vi "transmit_receive.vi"(4 "samples per readout":i32=5000, 5 "rotary queue":refnum<queue>, 6 "Continious mode":bool, 7 "Enable rotary encoder":bool, 8 "Waveform shift":waveform(dbl), 9 "Waveform drive":waveform(dbl), 10 "channel input for max readouts":T1, 11 "measurement queue":refnum<queue>) -> ()   [LabVIEW 2019]
doc: "This VI is responsible for collecting the data of the MPI experiment from the DAQ and it writes the data of the output waveforms to the DAQ. Generally, this VI can be operated in two modes: Continuous or non-continuous mode. In non-continuous mode, a finite number of samples is read from the ADC and a finite number of samples is written to the DAC. After playing these waveforms and acquiring the samples, the VI stops. The number of samples is determined by the product of \"samples per readout\" and the \"max readouts\" number passed to the VI via a channel structure. The latter allows to update the stopping condition while the acquisition is already running. Acquired data is written to a queue (has to be provided as an input) from which the main VI can then dequeue the readout buckets. Therefore, the sub-VI can be seen as the producer loop while the consumer loop is located in the main VI.\nIn continuous mode, a finite waveform sample is repeated over and over until the data acquisition reaches the set limit or it is stopped. \nInternally, the VI has three different DAQ tasks: Analog input acquisition, analog output generation and digital input acquisition. The analog input acquisition task is the \"master task\" and all other tasks are triggered when the analog data acquisition starts. \nMost of the DAQ settings are read from the global variables (including channel, channel type and sampling rate).\nThe rotary position is taken in the middle of the readout bucket. \nFor safety reasons, the VI ensures that zeros are written to the DAQ when stopping the VI properly."
uses:
  <extravilib>/ChannelInstances/Tag-dbl/))Channel.ctl
  <vilib>/DAQmx/write.llb/DAQmx Write (Analog 1D Wfm NChan NSamp).vi
  <vilib>/DAQmx/read.llb/DAQmx Read (Digital 1D U32 NChan 1Samp).vi
  <vilib>/DAQmx/read.llb/DAQmx Read (Analog 1D Wfm NChan NSamp).vi
  <vilib>/DAQmx/write.llb/DAQmx Write (Analog 2D DBL NChan NSamp).vi
  <vilib>/Waveform/WDTOps.llb/WDT Number of Waveform Samples DBL.vi
  global_variables.vi
  <vilib>/DAQmx/create/channels.llb/DAQmx Create Channel (AO-Voltage-Basic).vi
  <extravilib>/ChannelInstances/Tag-dbl/EndpointRead.vi
  <vilib>/DAQmx/configure/timing.llb/DAQmx Timing (Sample Clock).vi
  <vilib>/DAQmx/create/channels.llb/DAQmx Create Channel (AI-Voltage-Basic).vi
  <vilib>/DAQmx/configure/trigger.llb/DAQmx Start Trigger (None).vi
  <vilib>/DAQmx/configure/trigger.llb/DAQmx Start Trigger (Digital Edge).vi
  <vilib>/DAQmx/miscellaneous.llb/DAQmx Fill In Error Info.vi
  <vilib>/DAQmx/create/channels.llb/DAQmx Create Channel (DI-Digital Input).vi
  <extravilib>/ChannelInstances/Tag-dbl.lvlib
  <resource>/objmgr/daqmx.rc
panel:
  out "Homing & trigger readout":bool[](array[boolean])
  out "sample rate rotary encoder":dbl
  out "Boolean":bool
  out "Rotary aquisition stopped":bool
  out "rotary ro":i32
  out "Rotary encoder readout":bool[](array[boolean])
  out "Input waveforms":dynamicdata(graph)
  out "Transmit stopped":bool
  out "current readout no":i32
  out "RX":waveform(dbl)[](graph)
  out "Data aquisition stopped":bool
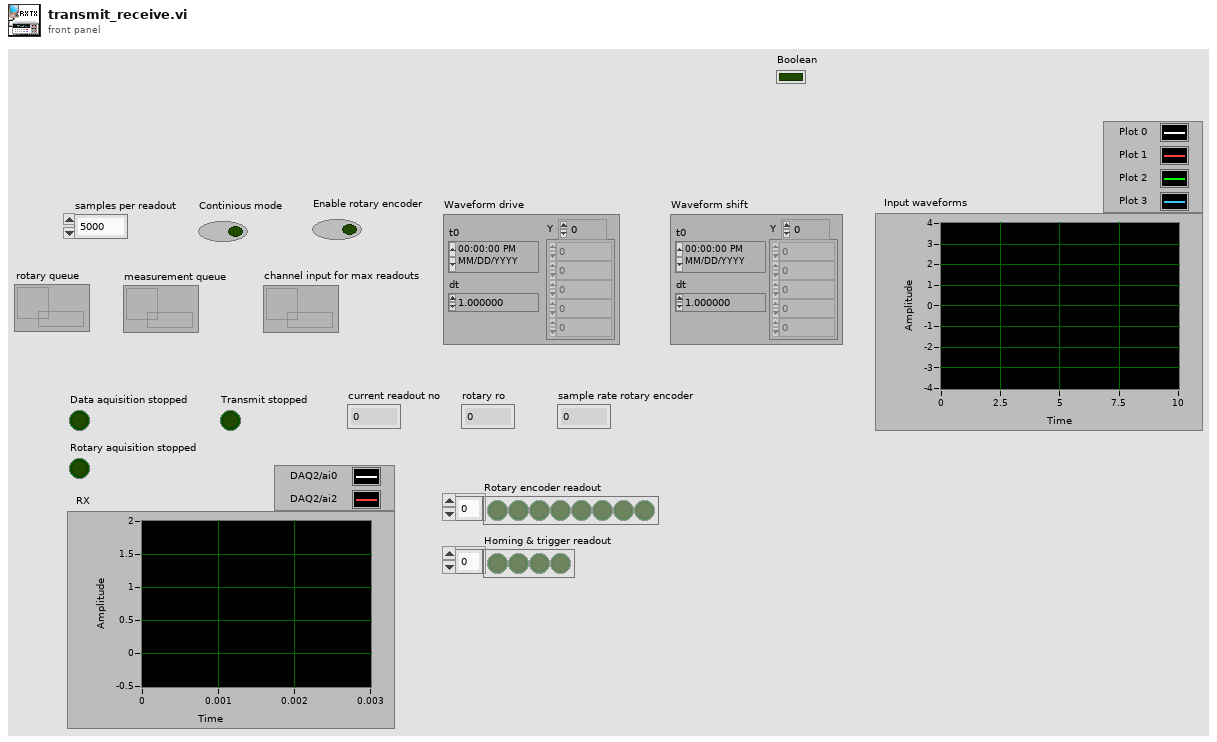
[diagram p1: front panel]
types:
  T1 = typedef "Tag-dbl.lvlib/))Channel.ctl" = refnum<queue>
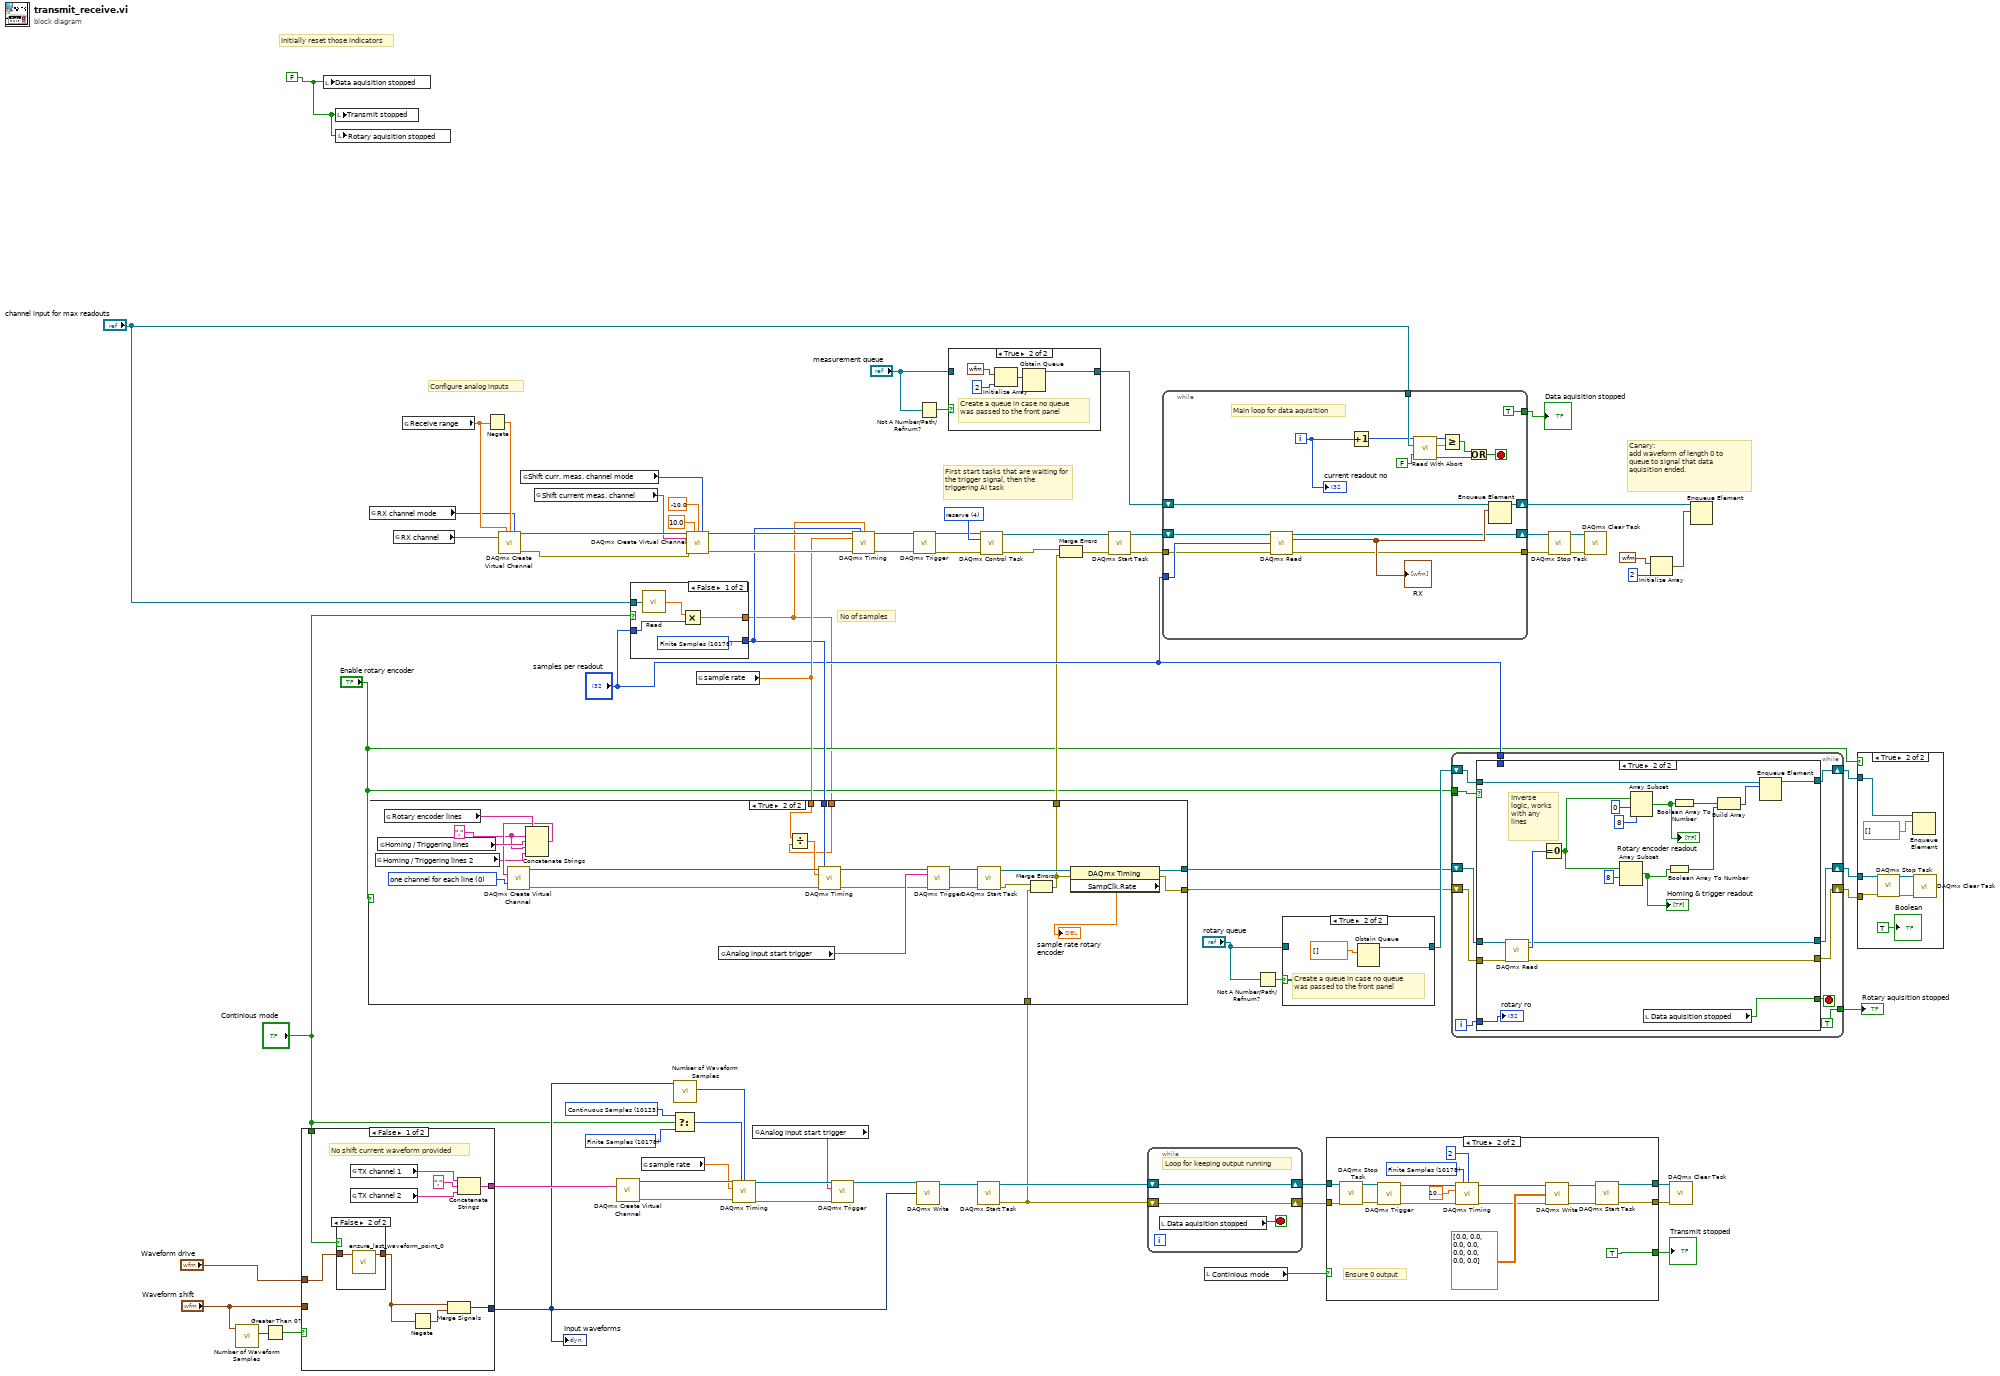
[diagram p0: block diagram]
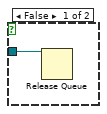
[diagram p2: hidden frame]
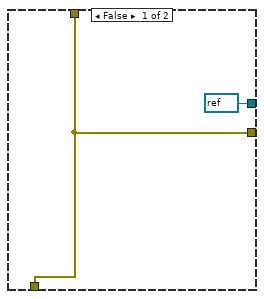
[diagram p3: hidden frame]
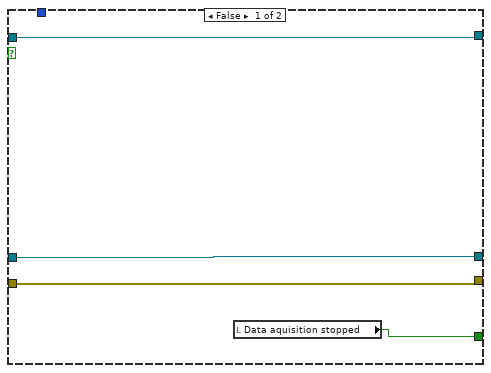
[diagram p5: hidden frame]
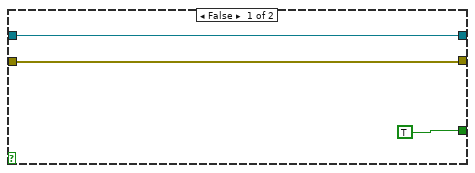
[diagram p6: hidden frame]
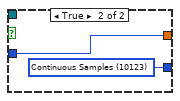
[diagram p7: hidden frame]
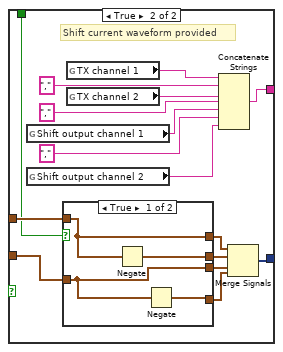
[diagram p10: hidden frame]
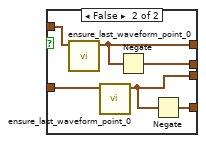
[diagram p11: hidden frame]
diagram:
  w33 = 4 items=["verify"=2, "reserve"=4, "commit"=3, "unreserve"=5, "abort"=6] ("action")
  w38 = 10178 items=["Finite Samples"=10178, "Continuous Samples"=10123, "Hardware Timed Single Point"=12522] ("sample mode")
  w39 = 10123 items=["Finite Samples"=10178, "Continuous Samples"=10123, "Hardware Timed Single Point"=12522] ("sample mode")
  w18 = FALSE ("Data aquisition stopped 2")
  # "First start tasks that are waiting for the trigger signal, then the triggering AI task"
  # "Configure analog inputs"
  # "Initially reset those indicators"
  # "Canary:\nadd waveform of length 0 to queue to signal that data aquisition ended."
  # "No of samples"
  n1 = call-poly <vilib>:"Number of Waveform Samples.vi"("waveform in"="Waveform shift") -> ("number of samples"=w2:i32)  [unwired: 8 in, 2 out]
  n2 = Greater Than 0?(x=w2) -> (x > 0?=w67:bool)
  n3 = case shown="False" w67 {
    tunnel: [w81 w106] -> w66
    tunnel: "Waveform shift" -> [_ w104]
    tunnel: "Waveform drive" -> [w86 w103]
    tunnel: [w87 w105] -> w45
    tunnel: "Continious mode" -> [w85 w101]
    frame False {
      # "No shift current waveform provided"
      n4 = case shown="False" w85 {
        tunnel: [w88 w90] -> w79
        tunnel: w86 -> [w88 w89]
        frame True {
        }
        frame False {
          n5 = call "ensure_last_waveform_point_0.vi"("Waveform in"=w89) -> ("Waveform out"=w90:waveform(dbl))  [unwired: 10 in]
        }
      }
      n6 = global read "global_variables.vi" "TX channel 1"() -> (w84:tag)
      n7 = global read "global_variables.vi" "TX channel 2"() -> (w83:tag)
      n8 = Negate(x=w79) -> (-x=w80:waveform(dbl))
      n9 = Merge Signals(w79, w80) -> (w87:dynamicdata)
      n10 = Concatenate Strings(w84, "," ("string"), w83) -> (w81:string)
    }
    frame True {
      # "Shift current waveform provided"
      n11 = global read "global_variables.vi" "Shift output channel 1"() -> (w99:tag)
      n12 = global read "global_variables.vi" "Shift output channel 2"() -> (w93:tag)
      n13 = case shown="True" w101 {
        tunnel: w104 -> [w108 w116]
        tunnel: [w108 w111] -> w95
        tunnel: w103 -> [w109 w115]
        tunnel: [w109 w114] -> w102
        tunnel: [w110 w113] -> w94
        tunnel: [w107 w112] -> w91
        frame True {
          n14 = Negate(x=w109) -> (-x=w110:waveform(dbl))
          n15 = Negate(x=w108) -> (-x=w107:waveform(dbl))
        }
        frame False {
          n16 = call "ensure_last_waveform_point_0.vi"("Waveform in"=w115) -> ("Waveform out"=w114:waveform(dbl))  [unwired: 10 in]
          n17 = call "ensure_last_waveform_point_0.vi"("Waveform in"=w116) -> ("Waveform out"=w111:waveform(dbl))  [unwired: 10 in]
          n18 = Negate(x=w114) -> (-x=w113:waveform(dbl))
          n19 = Negate(x=w111) -> (-x=w112:waveform(dbl))
        }
      }
      n20 = global read "global_variables.vi" "TX channel 1"() -> (w100:tag)
      n21 = global read "global_variables.vi" "TX channel 2"() -> (w98:tag)
      n22 = Concatenate Strings(w100, "," ("string"), w98, "," ("string"), w99, "," ("string"), w93) -> (w106:string)
      n23 = Merge Signals(w102, w94, w95, w91) -> (w105:dynamicdata)
    }
  }
  "Input waveforms" <- w45
  n24 = local write "Data aquisition stopped"(w18) -> ()
  n25 = local write "Transmit stopped"(w18) -> ()
  n26 = local write "Rotary aquisition stopped"(w18) -> ()
  n27 = global read "global_variables.vi" "RX channel mode"() -> (w42:i32)
  n28 = global read "global_variables.vi" "RX channel"() -> (w43:tag)
  n29 = global read "global_variables.vi" "Receive range"() -> (w55:dbl)
  n30 = Negate(x=w55) -> (-x=w54:dbl)
  n31 = call-poly <vilib>:"DAQmx Create Virtual Channel.vi"("maximum value"=w55, "minimum value"=w54, "input terminal configuration"=w42, "physical channels"=w43) -> ("task out"=w60:refnum<k21>, "error out"=w59:errorcluster)  [unwired: 10 in]
  n32 = global read "global_variables.vi" "Shift curr. meas. channel mode"() -> (w41:i32)
  n33 = global read "global_variables.vi" "Shift current meas. channel"() -> (w40:tag)
  n34 = call-poly <vilib>:"DAQmx Create Virtual Channel.vi"("physical channels"=w66) -> ("task out"=w72:refnum<k21>, "error out"=w69:errorcluster)  [unwired: 13 in]
  n35 = case shown="False" "Continious mode" {
    tunnel: [w121 w123] -> w25
    tunnel: "samples per readout" -> [w120 w122]
    tunnel: [w119 w122] -> w4
    tunnel: "channel input for max readouts" -> [w118 _]
    frame False {
      w121 = 10178 items=["Finite Samples"=10178, "Continuous Samples"=10123, "Hardware Timed Single Point"=12522] ("sample mode")
      n36 = call <extravilib>:"Read.vi"("channel"=w118) -> ("element"=w117:dbl)  [unwired: 1 in, 1 out]
      n37 = Multiply(x=w117, y=w120) -> (x*y=w119:dbl)
    }
    frame True {
      w123 = 10123 items=["Finite Samples"=10178, "Continuous Samples"=10123, "Hardware Timed Single Point"=12522] ("sample mode")
    }
  }
  n38 = global read "global_variables.vi" "sample rate"() -> (w46:dbl)
  n39 = Select(t=w39, s="Continious mode", f=w38) -> (s? t:f=w36:i32)
  n40 = call-poly <vilib>:"Number of Waveform Samples.vi"("waveform in"=w45) -> ("number of samples"=w44:i32)  [unwired: 8 in, 2 out]
  n41 = call-poly <vilib>:"DAQmx Create Virtual Channel.vi"("task in"=w60, "maximum value"=10.0, "minimum value"=-10.0, "input terminal configuration"=w41, "physical channels"=w40, "error in"=w59) -> ("task out"=w78:refnum<k21>, "error out"=w77:errorcluster)  [unwired: 8 in]
  n42 = global read "global_variables.vi" "sample rate"() -> (w34:dbl)
  n43 = call-poly <vilib>:"DAQmx Timing.vi"("task/channels in"=w72, "sample mode"=w36, "samples per channel"=w44, "rate"=w46, "error in"=w69) -> ("task out"=w71:refnum<k21>, "error out"=w70:errorcluster)  [unwired: 9 in]
  n44 = global read "global_variables.vi" "Analog input start trigger"() -> (w26:tag)
  n45 = call-poly <vilib>:"DAQmx Trigger.vi"("task/channels in"=w71, "source"=w26, "error in"=w70) -> ("task out"=w68:refnum<k21>)  [unwired: 11 in, 1 out]
  n46 = call-poly <vilib>:"DAQmx Timing.vi"("task/channels in"=w78, "sample mode"=w25, "samples per channel"=w4, "rate"=w34, "error in"=w77) -> ("task out"=w76:refnum<k21>, "error out"=w75:errorcluster)  [unwired: 9 in]
  n47 = call-poly <vilib>:"DAQmx Trigger.vi"("task/channels in"=w76, "error in"=w75) -> ("task out"=w31:refnum<k21>, "error out"=w32:errorcluster)  [unwired: 12 in]
  n48 = call-poly <vilib>:"DAQmx Write.vi"("task/channels in"=w68, "data"=w45) -> ("task out"=w48:refnum<k21>)  [unwired: 11 in, 2 out]
  n49 = Not A Number/Path/Refnum?(number/path/refnum="measurement queue") -> (NaN/Path/Refnum?=w63:bool)
  n50 = case shown="True" w63 {
    tunnel: "measurement queue" -> [w124 _]
    tunnel: [w124 w125] -> w62
    frame False {
    }
    frame True {
      # "Create a queue in case no queue was passed to the front panel"
      n51 = Initialize Array(waveform(dbl) {"t0"=timestamp(0 s since 1904-01-01), "dt"=1.0, "Y"=[]} ("Waveform"), 2 ("dimension size")) -> (w127:waveform(dbl)[])
      n52 = Obtain Queue(element data type=w127) -> (queue out=w125:refnum<queue>)  [unwired: 4 in, 2 out]
    }
  }
  n53 = call <vilib>:"DAQmx Start Task.vi"("task/channels in"=w48) -> ("task out"=w35:refnum<k21>, "error out"=w27:errorcluster)  [unwired: 13 in]
  n54 = case shown="True" "Enable rotary encoder" {
    tunnel: w34 -> [_ w143]
    tunnel: w27 -> [w129 w154]
    tunnel: w25 -> [_ w153]
    tunnel: [w129 w137] -> w20
    tunnel: [refnum<k21> refnum ("task out") w140] -> w14
    tunnel: [w129 w139] -> w9
    tunnel: w4 -> [_ w141]
    frame False {
    }
    frame True {
      w132 = "," ("string")
      w147 = 0 items=["one channel for each line", "one channel for all lines"] ("line grouping")
      n55 = global read "global_variables.vi" "Homing / Triggering lines 2"() -> (w131:tag)
      n56 = global read "global_variables.vi" "Homing / Triggering lines"() -> (w134:tag)
      n57 = global read "global_variables.vi" "Rotary encoder lines"() -> (w135:tag)
      n58 = Concatenate Strings(w135, w132, w134, w132, w131) -> (w133:string)
      n59 = call-poly <vilib>:"DAQmx Create Virtual Channel.vi"("lines"=w133, "line grouping"=w147) -> ("task out"=w150:refnum<k21>, "error out"=w151:errorcluster)  [unwired: 12 in]
      n60 = global read "global_variables.vi" "Analog input start trigger"() -> (w152:tag)
      n61 = Divide(x=w143, y=w141) -> (x/y=w142:dbl)
      n62 = call-poly <vilib>:"DAQmx Timing.vi"("task/channels in"=w150, "sample mode"=w153, "rate"=w142, "error in"=w151) -> ("task out"=w149:refnum<k21>, "error out"=w145:errorcluster)  [unwired: 10 in]
      n63 = call-poly <vilib>:"DAQmx Trigger.vi"("task/channels in"=w149, "source"=w152, "error in"=w145) -> ("task out"=w148:refnum<k21>, "error out"=w146:errorcluster)  [unwired: 11 in]
      n64 = call <vilib>:"DAQmx Start Task.vi"("task/channels in"=w148, "error in"=w146) -> ("task out"=w138:refnum<k21>, "error out"=w144:errorcluster)  [unwired: 12 in]
      n65 = Merge Errors(w144, w154) -> (w137:errorcluster)
      n66 = property class="DAQmx Timing"(reference=w138, error in=w137) -> (reference out=w140:refnum<k21>, error out=w139:errorcluster, "SampClk.Rate"=→"sample rate rotary encoder":dbl)
    }
  }
  n67 = call <vilib>:"DAQmx Control Task.vi"("task/channels in"=w31, "action"=w33, "error in"=w32) -> ("task out"=w30:refnum<k21>, "error out"=w29:errorcluster)  [unwired: 11 in]
  n68 = Merge Errors(w29, w20) -> (w28:errorcluster)
  n69 = call <vilib>:"DAQmx Start Task.vi"("task/channels in"=w30, "error in"=w28) -> ("task out"=w74:refnum<k21>, "error out"=w73:errorcluster)  [unwired: 12 in]
  n70 = while {
    shift-right: [w155] -> w53
    shift-left: w35 -> [w155]
    shift-right: [w156] -> w51
    shift-left: w27 -> [w156]
    stop <- w157 stop-if-true
    # "Loop for keeping output running"
    n71 = local read "Data aquisition stopped"() -> (w157:bool)
  }
  n72 = while {
    tunnel: w73 -> [w159]
    tunnel: "samples per readout" -> [w162]
    shift-right: [w171] -> w61
    shift-left: w62 -> [w172]
    tunnel: [TRUE] -> w64
    tunnel: "channel input for max readouts" -> [w170]
    shift-right: [w160] -> w5
    shift-left: w74 -> [w174]
    tunnel: [w158] -> w3
    i -> [w168]
    stop <- w163 stop-if-true
    # "Main loop for data aquisition"
    n73 = call-poly <vilib>:"DAQmx Read.vi"("task/channels in"=w174, "number of samples per channel"=w162, "error in"=w159) -> ("task out"=w160:refnum<k21>, "data"=w161:waveform(dbl)[], "error out"=w158:errorcluster)  [unwired: 10 in]
    "RX" <- w161
    n74 = Increment(x=w168) -> (x+1=w167:i32)
    n75 = call <extravilib>:"Read With Abort.vi"("abort"=FALSE, "channel"=w170) -> ("element"=w166:dbl, "aborted?"=w164:bool)  [unwired: 7 in, 1 out]
    n76 = Greater Or Equal?(x=w167, y=w166) -> (x >= y?=w165:bool)
    n77 = Or(x=w165, y=w164) -> (x .or. y?=w163:bool)
    n78 = Enqueue Element(queue=w172, element=w161) -> (queue out=w171:refnum<queue>)  [unwired: 2 in, 2 out]
    "current readout no" <- w168
  }
  "Data aquisition stopped" <- w64
  n79 = local read "Continious mode"() -> (w50:bool)
  n80 = Not A Number/Path/Refnum?(number/path/refnum="rotary queue") -> (NaN/Path/Refnum?=w15:bool)
  n81 = case shown="True" w15 {
    tunnel: "rotary queue" -> [w175 _]
    tunnel: [w175 w176] -> w17
    frame False {
    }
    frame True {
      # "Create a queue in case no queue was passed to the front panel"
      n82 = Obtain Queue(element data type=dbl[] []) -> (queue out=w176:refnum<queue>)  [unwired: 4 in, 2 out]
    }
  }
  n83 = case shown="True" w50 {
    tunnel: w53 -> [w180 w197]
    tunnel: [TRUE TRUE] -> w52
    tunnel: [w180 w192] -> w49
    tunnel: [w179 w186] -> w47
    tunnel: w51 -> [w179 w196]
    frame False {
    }
    frame True {
      w191 = 10178 items=["Finite Samples"=10178, "Continuous Samples"=10123, "Hardware Timed Single Point"=12522] ("sample mode")
      # "Ensure 0 output"
      n84 = call <vilib>:"DAQmx Stop Task.vi"("task/channels in"=w197, "error in"=w196) -> ("task out"=w195:refnum<k21>, "error out"=w194:errorcluster)  [unwired: 12 in]
      n85 = call-poly <vilib>:"DAQmx Trigger.vi"("task/channels in"=w195, "error in"=w194) -> ("task out"=w190:refnum<k21>, "error out"=w184:errorcluster)  [unwired: 12 in]
      n86 = call-poly <vilib>:"DAQmx Timing.vi"("task/channels in"=w190, "sample mode"=w191, "samples per channel"=2, "rate"=1000.0, "error in"=w184) -> ("task out"=w189:refnum<k21>, "error out"=w183:errorcluster)  [unwired: 9 in]
      n87 = call-poly <vilib>:"DAQmx Write.vi"("task/channels in"=w189, "data"=dbl[][] [[0.0, 0.0], [0.0, 0.0], [0.0, 0.0], [0.0, 0.0]], "error in"=w183) -> ("task out"=w193:refnum<k21>, "error out"=w182:errorcluster)  [unwired: 10 in, 1 out]
      n88 = call <vilib>:"DAQmx Start Task.vi"("task/channels in"=w193, "error in"=w182) -> ("task out"=w192:refnum<k21>, "error out"=w186:errorcluster)  [unwired: 12 in]
    }
  }
  "Transmit stopped" <- w52
  n89 = while {
    shift-right: [w207] -> w13
    shift-left: w14 -> [w208]
    shift-right: [w200] -> w12
    shift-left: w9 -> [w201]
    shift-right: [w202] -> w10
    shift-left: w17 -> [w203]
    tunnel: "samples per readout" -> [w199]
    tunnel: [TRUE ("Boolean")] -> w11
    tunnel: [w198] -> _
    tunnel: "Enable rotary encoder" -> [w198]
    i -> [w205]
    stop <- w206 stop-if-true
    n90 = case shown="True" w198 {
      tunnel: w208 -> [w211 w230]
      tunnel: [w211 w218] -> w207
      tunnel: [w209 w222] -> w206
      tunnel: w205 -> [_ w228]
      tunnel: w203 -> [w212 w227]
      tunnel: [w212 w226] -> w202
      tunnel: w201 -> [w210 w224]
      tunnel: [w210 w217] -> w200
      tunnel: w199 -> [_ _]
      frame False {
        n91 = local read "Data aquisition stopped"() -> (w209:bool)
      }
      frame True {
        # "Inverse logic, works with any lines"
        n92 = call-poly <vilib>:"DAQmx Read.vi"("task/channels in"=w230, "error in"=w224) -> ("task out"=w218:refnum<k21>, "data"=w229:u32[], "error out"=w217:errorcluster)  [unwired: 11 in]
        n93 = Equal To 0?(x=w229) -> (x = 0?=w216:bool[])
        n94 = Array Subset(array=w216, index=8) -> (w214:bool[])  [unwired: 1 in]
        "Homing & trigger readout" <- w214
        n95 = Array Subset(array=w216, index=0, length=8) -> (w221:bool[])
        "Rotary encoder readout" <- w221
        n96 = local read "Data aquisition stopped"() -> (w222:bool)
        n97 = Boolean Array To Number(Boolean array=w214) -> (number=w213:u32)
        n98 = Boolean Array To Number(Boolean array=w221) -> (number=w223:u32)
        n99 = Build Array(w223, w213) -> (w225:u32[])
        n100 = Enqueue Element(queue=w227, element=w225) -> (queue out=w226:refnum<queue>)  [unwired: 2 in, 2 out]
        "rotary ro" <- w228
      }
    }
  }
  "Rotary aquisition stopped" <- w11
  n101 = call <vilib>:"DAQmx Stop Task.vi"("task/channels in"=w5, "error in"=w3) -> ("task out"=w7:refnum<k21>, "error out"=w6:errorcluster)  [unwired: 12 in]
  n102 = call <vilib>:"DAQmx Clear Task.vi"("task in"=w7, "error in"=w6) -> ()  [unwired: 13 in, 1 out]
  n103 = Initialize Array(waveform(dbl) {"t0"=timestamp(0 s since 1904-01-01), "dt"=1.0, "Y"=[]} ("Waveform"), 2 ("dimension size")) -> (w22:waveform(dbl)[])
  n104 = call <vilib>:"DAQmx Clear Task.vi"("task in"=w49, "error in"=w47) -> ()  [unwired: 13 in, 1 out]
  n105 = Enqueue Element(queue=w61, element=w22) -> ()  [unwired: 2 in, 3 out]
  n106 = case shown="True" "Enable rotary encoder" {
    tunnel: w13 -> [_ w236]
    tunnel: w12 -> [_ w233]
    tunnel: w10 -> [w231 w238]
    frame False {
      n107 = Release Queue(queue=w231) -> ()  [unwired: 2 in, 3 out]
    }
    frame True {
      n108 = call <vilib>:"DAQmx Stop Task.vi"("task/channels in"=w236, "error in"=w233) -> ("task out"=w235:refnum<k21>, "error out"=w234:errorcluster)  [unwired: 12 in]
      n109 = Enqueue Element(queue=w238, element=dbl[] []) -> ()  [unwired: 2 in, 3 out]
      n110 = call <vilib>:"DAQmx Clear Task.vi"("task in"=w235, "error in"=w234) -> ()  [unwired: 13 in, 1 out]
      "Boolean" <- TRUE ("Boolean")
    }
  }
